vi "Read tolerance limits params.vi"(7 "JSON Read":T5, 8 "error in (no error)":errorcluster, 9 "MeasurementListBox":refnum<vi>, 10 "Part Name":string, 11 "Edit Tolerance Settings Cluster":T1) -> (0 "error out":errorcluster, 2 "Number of\nMeasurements":u8, 3 "Edit Tolerance Settings Cluster 2":T1)   [LabVIEW 2019, in "ZenGage v3.0 UI.lvclass"]
uses:
  ZenGage v3.0 UI.lvclass
  Type Definitions/JSON Read/UI JSON read cluster.ctl
  Type Definitions/General/JSONRead.ctl
  Type Definitions/Edit tolerance settings/Rack Selection.ctl
  <vilib>/Utility/miscctls.llb/LVPoint32TypeDef.ctl
  Type Definitions/Edit tolerance settings/Edit Tolerance Input.ctl
  Type Definitions/Edit tolerance settings/Edit Tolerance Overall Cluster.ctl
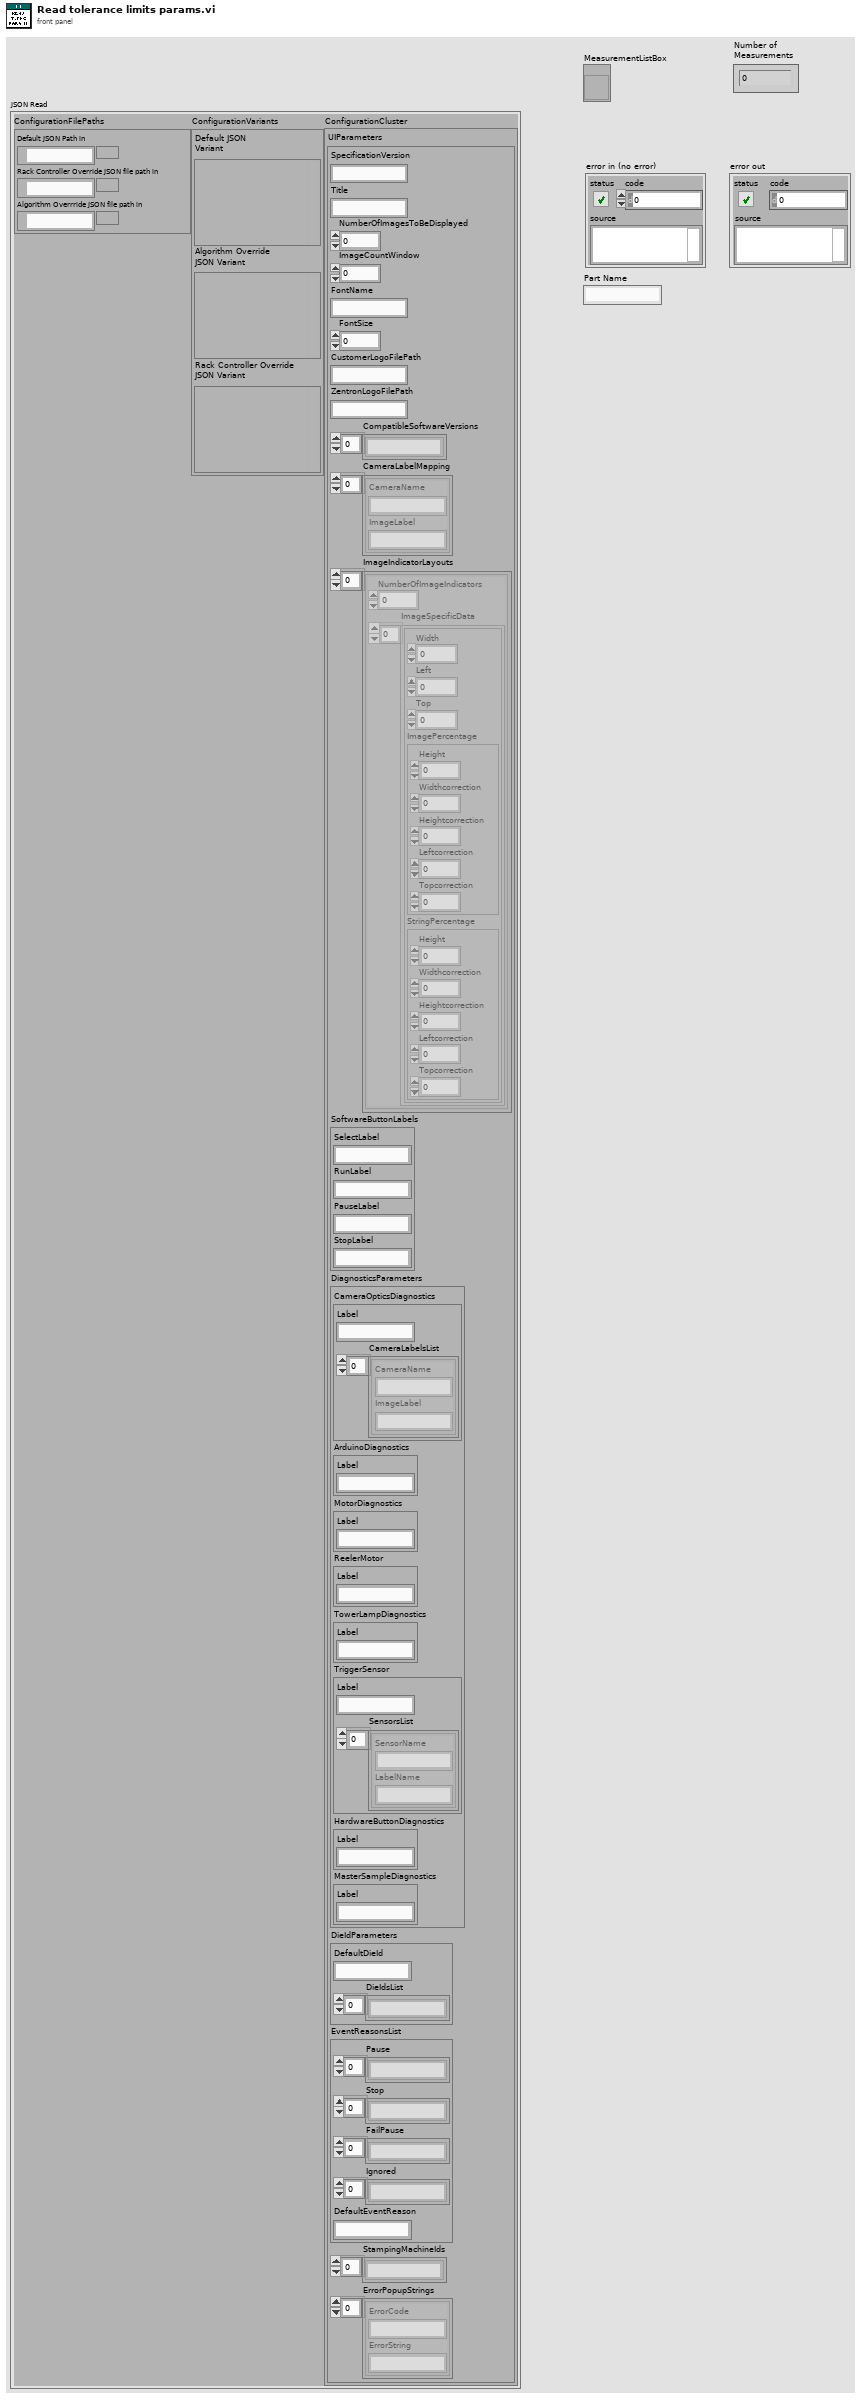
[diagram p1: front panel]
types:
  T1 = typedef "ZenGage v3.0 UI.lvclass/Edit Tolerance Overall Cluster.ctl" = cluster{"Input ListBox":T2, "Saved?":bool, "IsETLSelected":bool, "IsPartSelected":bool}
  T2 = typedef "ZenGage v3.0 UI.lvclass/Edit Tolerance Input.ctl" = cluster{"Measurement Values":string[][], "Cluster of Limits":cluster{"LSL":dbl, "USL":dbl, "LCL":dbl, "UCL":dbl}, "Rack Selection":T3, "M and N Array":cluster{"M1":u64, "M2":u64, "N1":u64, "N2":u64}[], "Ticked Measurement Index":u32[], "Measurements Enabled":bool[], "Current Active Position":T4, "Current ticked measurement":dbl}
  T3 = typedef "ZenGage v3.0 UI.lvclass/Rack Selection.ctl" = enum16{"Both Racks", "Rack 2", "Rack 1"}
  T4 = typedef "LVPoint32TypeDef.ctl" = cluster{"Horizontal":i32, "Vertical":i32}
  T5 = typedef "ZenGage v3.0 UI.lvclass/JSONRead.ctl" = cluster{"ConfigurationFilePaths":cluster{"Default JSON Path in":path, "Rack Controller Override JSON file path in":path, "Algorithm Overrride JSON file path in ":path}, "ConfigurationVariants":cluster{"Default JSON \nVariant":variant, "Algorithm Override\nJSON Variant":variant, "Rack Controller Override\nJSON Variant":variant}, "ConfigurationCluster":T6}
  T6 = typedef "ZenGage v3.0 UI.lvclass/UI JSON read cluster.ctl" = cluster{"UIParameters":cluster{"SpecificationVersion":string, "Title":string, "NumberOfImagesToBeDisplayed":dbl, "ImageCountWindow":dbl, "FontName":string, "FontSize":dbl, "CustomerLogoFilePath":string, "ZentronLogoFilePath":string, "CompatibleSoftwareVersions":string[], "CameraLabelMapping":cluster{"CameraName":string, "ImageLabel":string}[], "ImageIndicatorLayouts":cluster{"NumberOfImageIndicators":dbl, "ImageSpecificData":cluster{"Width":dbl, "Left":dbl, "Top":dbl, "ImagePercentage":cluster{"Height":dbl, "Widthcorrection":i64, "Heightcorrection":i64, "Leftcorrection":dbl, "Topcorrection":dbl}, "StringPercentage":cluster{"Height":dbl, "Widthcorrection":i64, "Heightcorrection":dbl, "Leftcorrection":dbl, "Topcorrection":dbl}}[]}[], "SoftwareButtonLabels":cluster{"SelectLabel":string, "RunLabel":string, "PauseLabel":string, "StopLabel":string}, "DiagnosticsParameters":cluster{"CameraOpticsDiagnostics":cluster{"Label":string, "CameraLabelsList":cluster{"CameraName":string, "ImageLabel":string}[]}, "ArduinoDiagnostics":cluster{"Label":string}, "MotorDiagnostics":cluster{"Label":string}, "ReelerMotor":cluster{"Label":string}, "TowerLampDiagnostics":cluster{"Label":string}, "TriggerSensor":cluster{"Label":string, "SensorsList":cluster{"SensorName":string, "LabelName":string}[]}, "HardwareButtonDiagnostics":cluster{"Label":string}, "MasterSampleDiagnostics":cluster{"Label":string}}, "DieIdParameters":cluster{"DefaultDieId":string, "DieIdsList":string[]}, "EventReasonsList":cluster{"Pause":string[], "Stop":string[], "FailPause":string[], "Ignored":string[], "DefaultEventReason":string}, "StampingMachineIds":string[], "ErrorPopupStrings":cluster{"ErrorCode":string, "ErrorString":string}[]}}
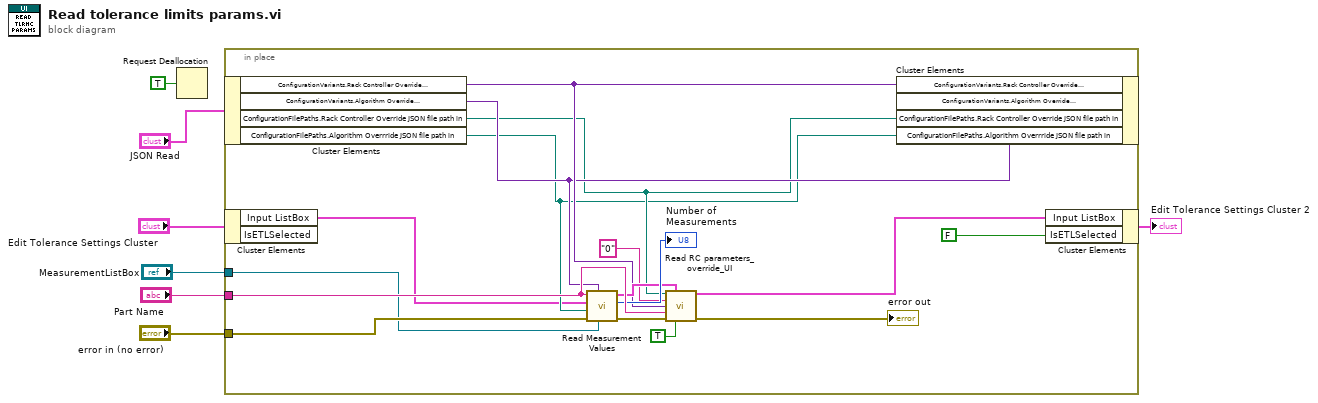
[diagram p0: block diagram]
diagram:
  n1 = Request Deallocation(TRUE ("flag")) -> ()
  n2 = in-place {
    in-place-border: "Part Name" -> [w22]
    in-place-border: "error in (no error)" -> [w12]
    in-place-border: "MeasurementListBox" -> [w9]
    n3 = in-place-cluster #1("JSON Read") -> ("ConfigurationVariants.Rack Controller Override\nJSON Variant"=w16:variant, "ConfigurationVariants.Algorithm Override\nJSON Variant"=w15:variant, "ConfigurationFilePaths.Rack Controller Override JSON file path in"=w14:path, "ConfigurationFilePaths.Algorithm Overrride JSON file path in"=w13:path)
    n4 = in-place-cluster #2("Edit Tolerance Settings Cluster") -> ("Input ListBox"=w11:T2)  [unwired: 1 out]
    n5 = call "Read Measurement Values.vi"("MeasurementListBox"=w9, "Algo Override\nJSON Variant in"=w15, "error in"=w12, "Read Edit Tolerance \nOverride JSON"=w13, "Input ListBox Cluster"=w11, "Part Name in"=w22) -> ("error out"=w20:errorcluster, "Number of\nMeasurements"=→"Number of\nMeasurements":u8, "ListBox Cluster out"=w19:T2)  [unwired: 3 in]
    n6 = call "Read RC parameters_override_UI.vi"("JSON FilePath"=w14, "ListBox Cluster"=w19, "Rack Id"="0", "Variant"=w16, "Part Name"=w22, "error in (no error)"=w20, "Variant?"=TRUE) -> ("Output Edit Tolerance cluster"=w8:T2, "error out"=→"error out":errorcluster)  [unwired: 6 in, 1 out]
    n7 = in-place-cluster #1("ConfigurationVariants.Rack Controller Override\nJSON Variant"=w16, "ConfigurationVariants.Algorithm Override\nJSON Variant"=w15, "ConfigurationFilePaths.Rack Controller Override JSON file path in"=w14, "ConfigurationFilePaths.Algorithm Overrride JSON file path in"=w13) -> ()  [unwired: 1 out]
    n8 = in-place-cluster #2("Input ListBox"=w8, "IsETLSelected"=FALSE ("General.Edit Tolerance Selected")) -> (→"Edit Tolerance Settings Cluster 2":T1)
  }
